vi "To String (Object).vi"(6 "pretty print? (T)":bool=TRUE, 7 "enable LabVIEW extensions? (T)":bool=TRUE, 8 "error in (no error)":errorcluster, 10 "indent":i32, 11 "JSON Value in":refnum<class "JSON Value.lvclass">) -> (0 "error out":errorcluster, 3 "String":string)   [LabVIEW 2017, in "JSON Value.lvclass"]
doc: "Flattens the given JSON data to a string."
uses:
  JSON Value.lvclass
  JSON Value.lvclass/JSON Value.ctl
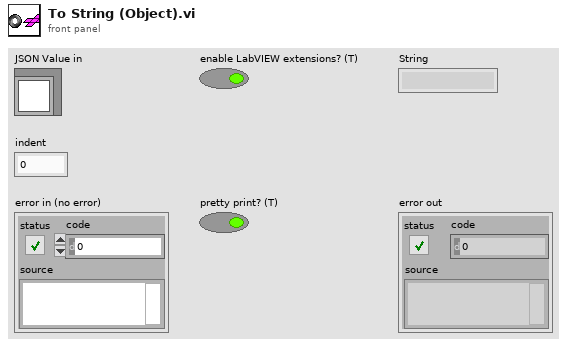
[diagram p1: front panel]
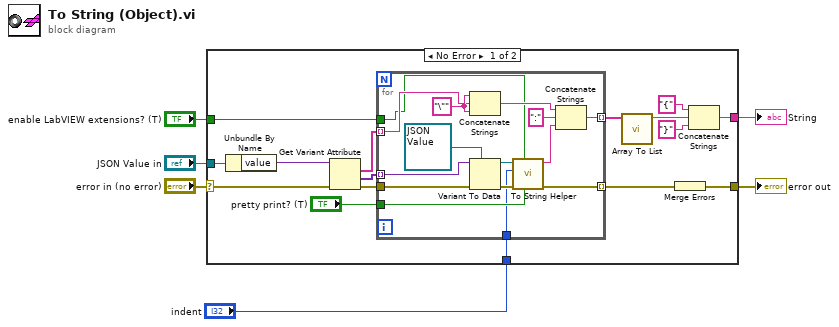
[diagram p0: block diagram]
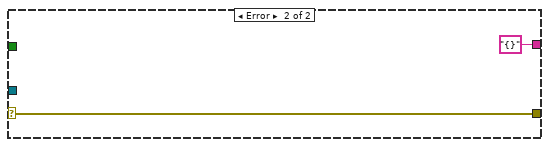
[diagram p2: hidden frame]
diagram:
  n1 = case shown="No Error" "error in (no error)" {
    selector: "error in (no error)" -> [w15 w38]
    tunnel: "JSON Value in" -> [w22 _]
    tunnel: [w18 "{}"] -> w5
    tunnel: [w12 w38] -> w3
    tunnel: "enable LabVIEW extensions? (T)" -> [w9 _]
    tunnel: "indent" -> [w7 _]
    frame No Error {
      n2 = Unbundle By Name(w22) -> ("value"=w21:variant)
      n3 = Get Variant Attribute(Variant=w21, error in=w15) -> (names=w20:string[], values=w19:variant[], error out=w14:errorcluster)  [unwired: 2 in, 1 out]
      n4 = for {
        tunnel: w20 -> [w33] mode=indexing
        tunnel: w19 -> [w37] mode=indexing
        tunnel: [w35] -> w17 mode=indexing
        tunnel: w14 -> [w29]
        tunnel: [w27] -> w13 mode=indexing
        tunnel: w9 -> [w26]
        tunnel: "pretty print? (T)" -> [w24]
        tunnel: w7 -> [w23]
        w34 = "\"" ("string")
        n5 = Concatenate Strings(w34, w33, w34) -> (w32:string)
        n6 = Variant To Data(error in=w29, type=refnum<class "JSON Value.lvclass"> refnum ("JSON Object in"), Variant=w37) -> (data=w31:refnum<class "JSON Value.lvclass">, error out=w28:errorcluster)
        n7 = call "To String Helper.vi"("pretty print? (T)"=w24, "enable LabVIEW extensions? (T)"=w26, "error in (no error)"=w28, "indent"=w23, "JSON Value in"=w31) -> ("error out"=w27:errorcluster, "String"=w30:string)  [unwired: 5 in]
        n8 = Concatenate Strings(w32, ":" ("string"), w30) -> (w35:string)
      }
      n9 = call "Array To List.vi"("Array"=w17) -> ("String"=w16:string)  [unwired: 10 in]
      n10 = Merge Errors(w13) -> (w12:errorcluster)
      n11 = Concatenate Strings("{" ("string"), w16, "}" ("string")) -> (w18:string)
    }
    frame Error {
    }
  }
  "String" <- w5
  "error out" <- w3
